vi "count_r2.vi"() -> ()   [LabVIEW 2015]
uses:
  <vilib>/myRIO/Instrument Drivers/Onboard IO/PWM/typedefs/PWM Reference.ctl
  <vilib>/myRIO/Common/Instrument Driver Framework/Utilities/typedefs/myRIO Generic Hardware Reference.ctl
  <vilib>/myRIO/Common/Instrument Driver Framework/Utilities/typedefs/Hardware Version Enum.ctl
  <vilib>/myRIO/Common/Instrument Driver Framework/Utilities/typedefs/myRIO v1.0 Reference.ctl
  <vilib>/myRIO/Common/Instrument Driver Framework/Utilities/typedefs/Generic FPGA Reference.ctl
  <vilib>/myRIO/Common/Instrument Driver Framework/myRIO v1.0/PWM/typedefs/PWM Channels Enum.ctl
  <vilib>/myRIO/Instrument Drivers/Onboard IO/PWM/typedefs/PWM Configuration.ctl
  <vilib>/userdefined/High Color/nirio_resource_hc.ctl
  <vilib>/myRIO/Common/Instrument Driver Framework/myRIO v1.0/PWM/vis/myRIO v1.1 Open PWM.vi
  <vilib>/myRIO/Common/Instrument Driver Framework/Utilities/vis/Validate Channels.vi
  <vilib>/myRIO/Common/Instrument Driver Framework/myRIO v1.0/PWM/vis/myRIO v1.0 Reserve PWM.vi
  <vilib>/myRIO/Instrument Drivers/Onboard IO/PWM/vis/Set Duty Cycle and Frequency.vi
  <vilib>/myRIO/Common/Instrument Driver Framework/myRIO v1.0/PWM/vis/myRIO v1.0 Build MUX Configuration PWM.vi
  <vilib>/myRIO/Common/Instrument Driver Framework/myRIO v1.0/Resource Manager/vis/myRIO v1.0 Reserve Channel List.vi
  <vilib>/myRIO/Common/Instrument Driver Framework/myRIO v1.0/Resource Manager/vis/myRIO v1.0 Create Configuration List.vi
  <vilib>/myRIO/Common/Instrument Driver Framework/myRIO v1.0/Resource Manager/vis/myRIO v1.0 Reserve Channel.vi
  <vilib>/myRIO/Common/Instrument Driver Framework/myRIO v1.0/Resource Manager/vis/myRIO v1.0 Unreserve Channel.vi
  <vilib>/myRIO/Common/Instrument Driver Framework/myRIO v1.0/Resource Manager/vis/myRIO v1.0 Build Mutex Name.vi
  <vilib>/FPGAPlugInAG/myRIO-1900/niLvFpga_Open_myRIO-1900.vi
  <vilib>/rvi/interface/common/dynamic/niFpgaDynamicAddResources.vi
  <vilib>/myRIO/Common/Instrument Driver Framework/Utilities/vis/FPGA Ref Manager.vi
  <vilib>/Utility/error.llb/Error Cluster From Error Code.vi
  <vilib>/myRIO/Common/Instrument Driver Framework/Utilities/vis/Ref Counter.vi
  <vilib>/rvi/errors/niLvFpgaAdjustHostInterfaceError.vi
  <vilib>/Utility/VariantDataType/GetNumericInfo.vi
  <vilib>/myRIO/Common/Instrument Driver Framework/myRIO v1.0/myRIO v1.1 Open.vi
  <vilib>/myRIO/Common/Instrument Driver Framework/Utilities/vis/IO Manager.vi
  <vilib>/myRIO/Common/Instrument Driver Framework/Utilities/vis/Configuration Manager.vi
  <vilib>/myRIO/Common/Instrument Driver Framework/myRIO v1.0/Resource Manager/vis/myRIO v1.0 Configure IO.vi
  <vilib>/myRIO/Common/Instrument Driver Framework/myRIO v1.0/myRIO v1.0 Close.vi
  <vilib>/myRIO/Common/Instrument Driver Framework/myRIO v1.0/PWM/vis/myRIO v1.0 Write PWM.vi
  <vilib>/rvi/interface/nirviOpenFPGA/nirviOpenFPGA.xnode
  FPGA Bitfiles/NavigationProjec_FPGATarget2_FPGAMainNavigati_PWPHW8gwDxI.lvbitx
  <vilib>/rvi/interface/nirviReadWriteControl/nirviReadWriteControl.xnode
  <vilib>/myRIO/Instrument Drivers/Onboard IO/PWM/vis/myRIO PWM Open.xnode
  <vilib>/myRIO/Instrument Drivers/Onboard IO/PWM/PWM.lvlib
  <vilib>/myRIO/Instrument Drivers/Utilities/Utilities.lvlib
  NiFpgaLv.dll
  <vilib>/rvi/interface/Simulation/niFpgaSimulationCallBeginRW.vi
panel:
  out "X Pos Lin Estimate":dbl
  out "Delta Lin Distance (ft)":dbl
  out "X Position Estimate":dbl
  out "Delta Distance (ft)":dbl
  out "heading degrees":dbl
  out "avg 456":dbl
  out "avg 123":dbl
  out "y position":dbl
  out "x position":dbl
  in  "start y":dbl=3.0
  in  "start x":dbl=1.0
  out "Delta Encoder Array":u32[](array[numeric])
  out "Robot Heading":dbl
  out "Current Encoder Array":u32[](array[numeric])
  out "Initial Encoder Array":u32[](array[numeric])
  in  "Encoder Reset":bool
  in  "master motor on switch":bool
  out "L Min Linear Velocity (ft/s) 2":dbl
  out "R Min Linear Velocity (ft/s)  2":dbl
  in  "Goal Y":dbl=3.0 format="%#_13g"
  in  "Goal X":dbl=20.0 format="%#_13g"
  out "x+y":dbl
  out "SYS.SELECTA":u8 format="%08b"
  out "ENC.B_c.CNTR":i32
  out "ENC.B_b.CNTR":i32
  out "ENC.B_a.CNTR":i32
  out "ENC.A_c.CNTR":i32
  out "ENC.A_b.CNTR":i32
  out "ENC.A_a.CNTR":i32
  out "Boolean":bool
  in  "R Desired Input Velocity (ft/s) 2":dbl(knob) scale=-4.0..4.0
  in  "front enable":bool
  in  "mid enable":bool
  in  "Rear enable":bool
  in  "Sync L -> R":bool
  in  "R Min Linear Velocity (ft/s)":dbl=-2.0 format="%#_13g"
  in  "R Max Linear Velocity (ft/s)":dbl=2.0 format="%#_13g"
  out "Rotational Velocity (RPS)":dbl
  in  "L Min Linear Velocity (ft/s)":dbl=-2.0 format="%#_13g"
  in  "L Max Linear Velocity (ft/s)":dbl=2.0 format="%#_13g"
  out "Current Rot Velocity (rot/s)":T1(graph)
  in  "L Desired Input Velocity (ft/s)":dbl(knob) scale=-4.0..4.0
  # "Motor Control Parameters"
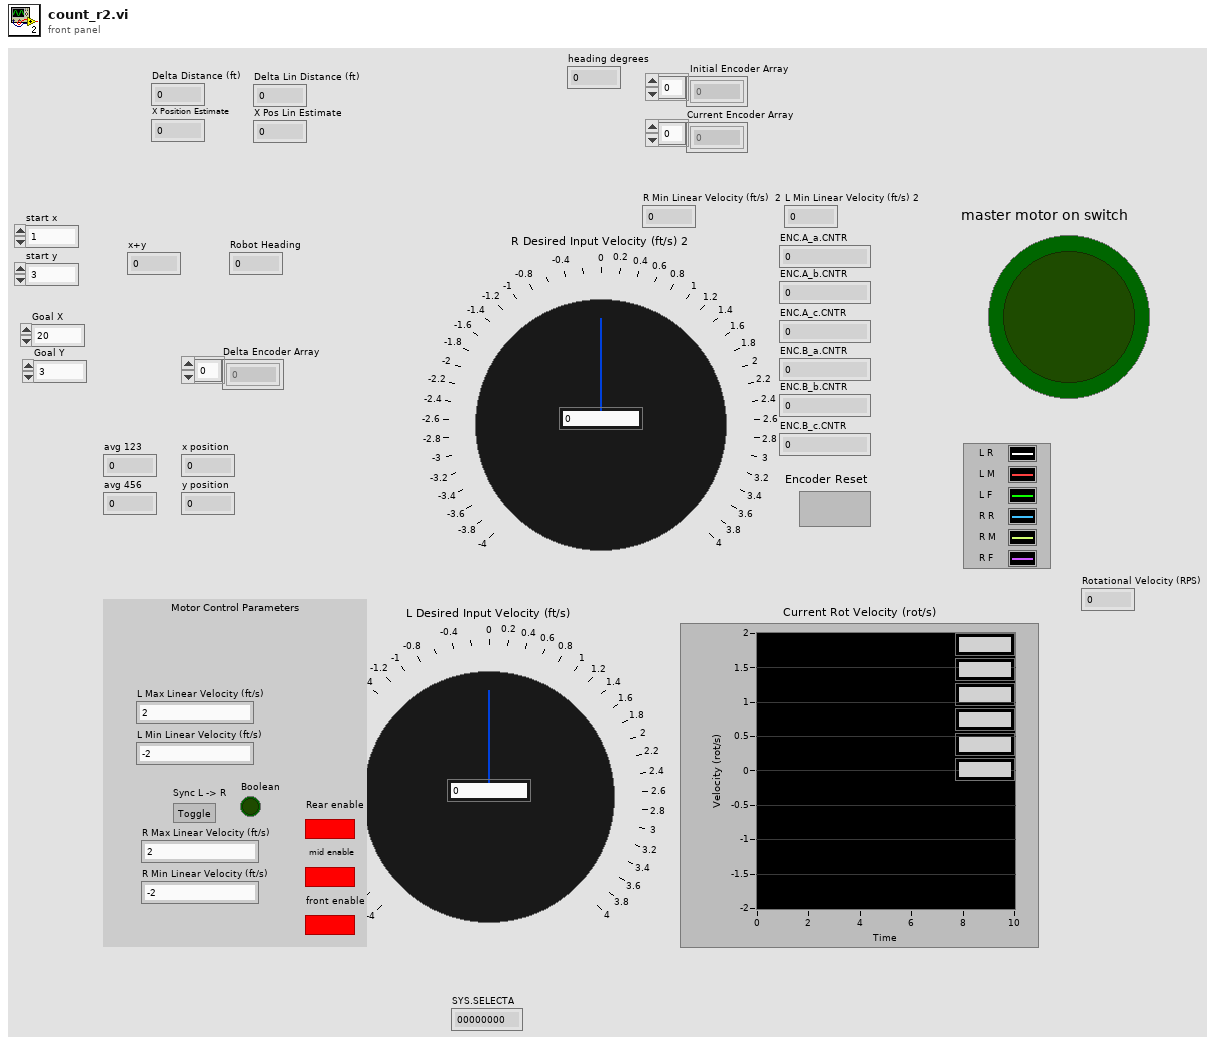
[diagram p1: front panel]
types:
  T1 = cluster{"Rotational Velocity (RPS)":dbl, "Rotational Velocity (RPS)":dbl, "Rotational Velocity (RPS)":dbl, "Rotational Velocity (RPS)":dbl, "Rotational Velocity (RPS)":dbl, "Rotational Velocity (RPS)":dbl}
  T2 = typedef "nirio_resource_hc.ctl" = tag
  T3 = typedef "Hardware Version Enum.ctl" = enum16{"Unknown", "myRIO-1900", "myRIO-1950", "roboRIO"}
  T4 = typedef "PWM.lvlib/PWM Reference.ctl" = cluster{"myRIO Reference":T5, "PWM Channels Enum":T8, "PWM Configuration":T9}
  T5 = typedef "myRIO Generic Hardware Reference.ctl" = cluster{"myRIO Model":T3, "myRIO Hardware Reference":T6}
  T6 = typedef "myRIO v1.0 Reference.ctl" = cluster{"Generic FPGA Reference":T7, "Allow multiple opens":bool}
  T7 = typedef "Generic FPGA Reference.ctl" = refnum<k20>
  T8 = typedef "PWM Channels Enum.ctl" = enum16{"Not Connected", "C/PWM0", "C/PWM1", "A/PWM0", "A/PWM1", "A/PWM2", "B/PWM0", "B/PWM1", "B/PWM2", "PWM/PWM0", "PWM/PWM1", "PWM/PWM2", "PWM/PWM3", "PWM/PWM4", "PWM/PWM5", "PWM/PWM6", "PWM/PWM7", "PWM/PWM8", "PWM/PWM9"}
  T9 = typedef "PWM.lvlib/PWM Configuration.ctl" = cluster{"Frequency":dbl, "Duty Cycle":dbl}
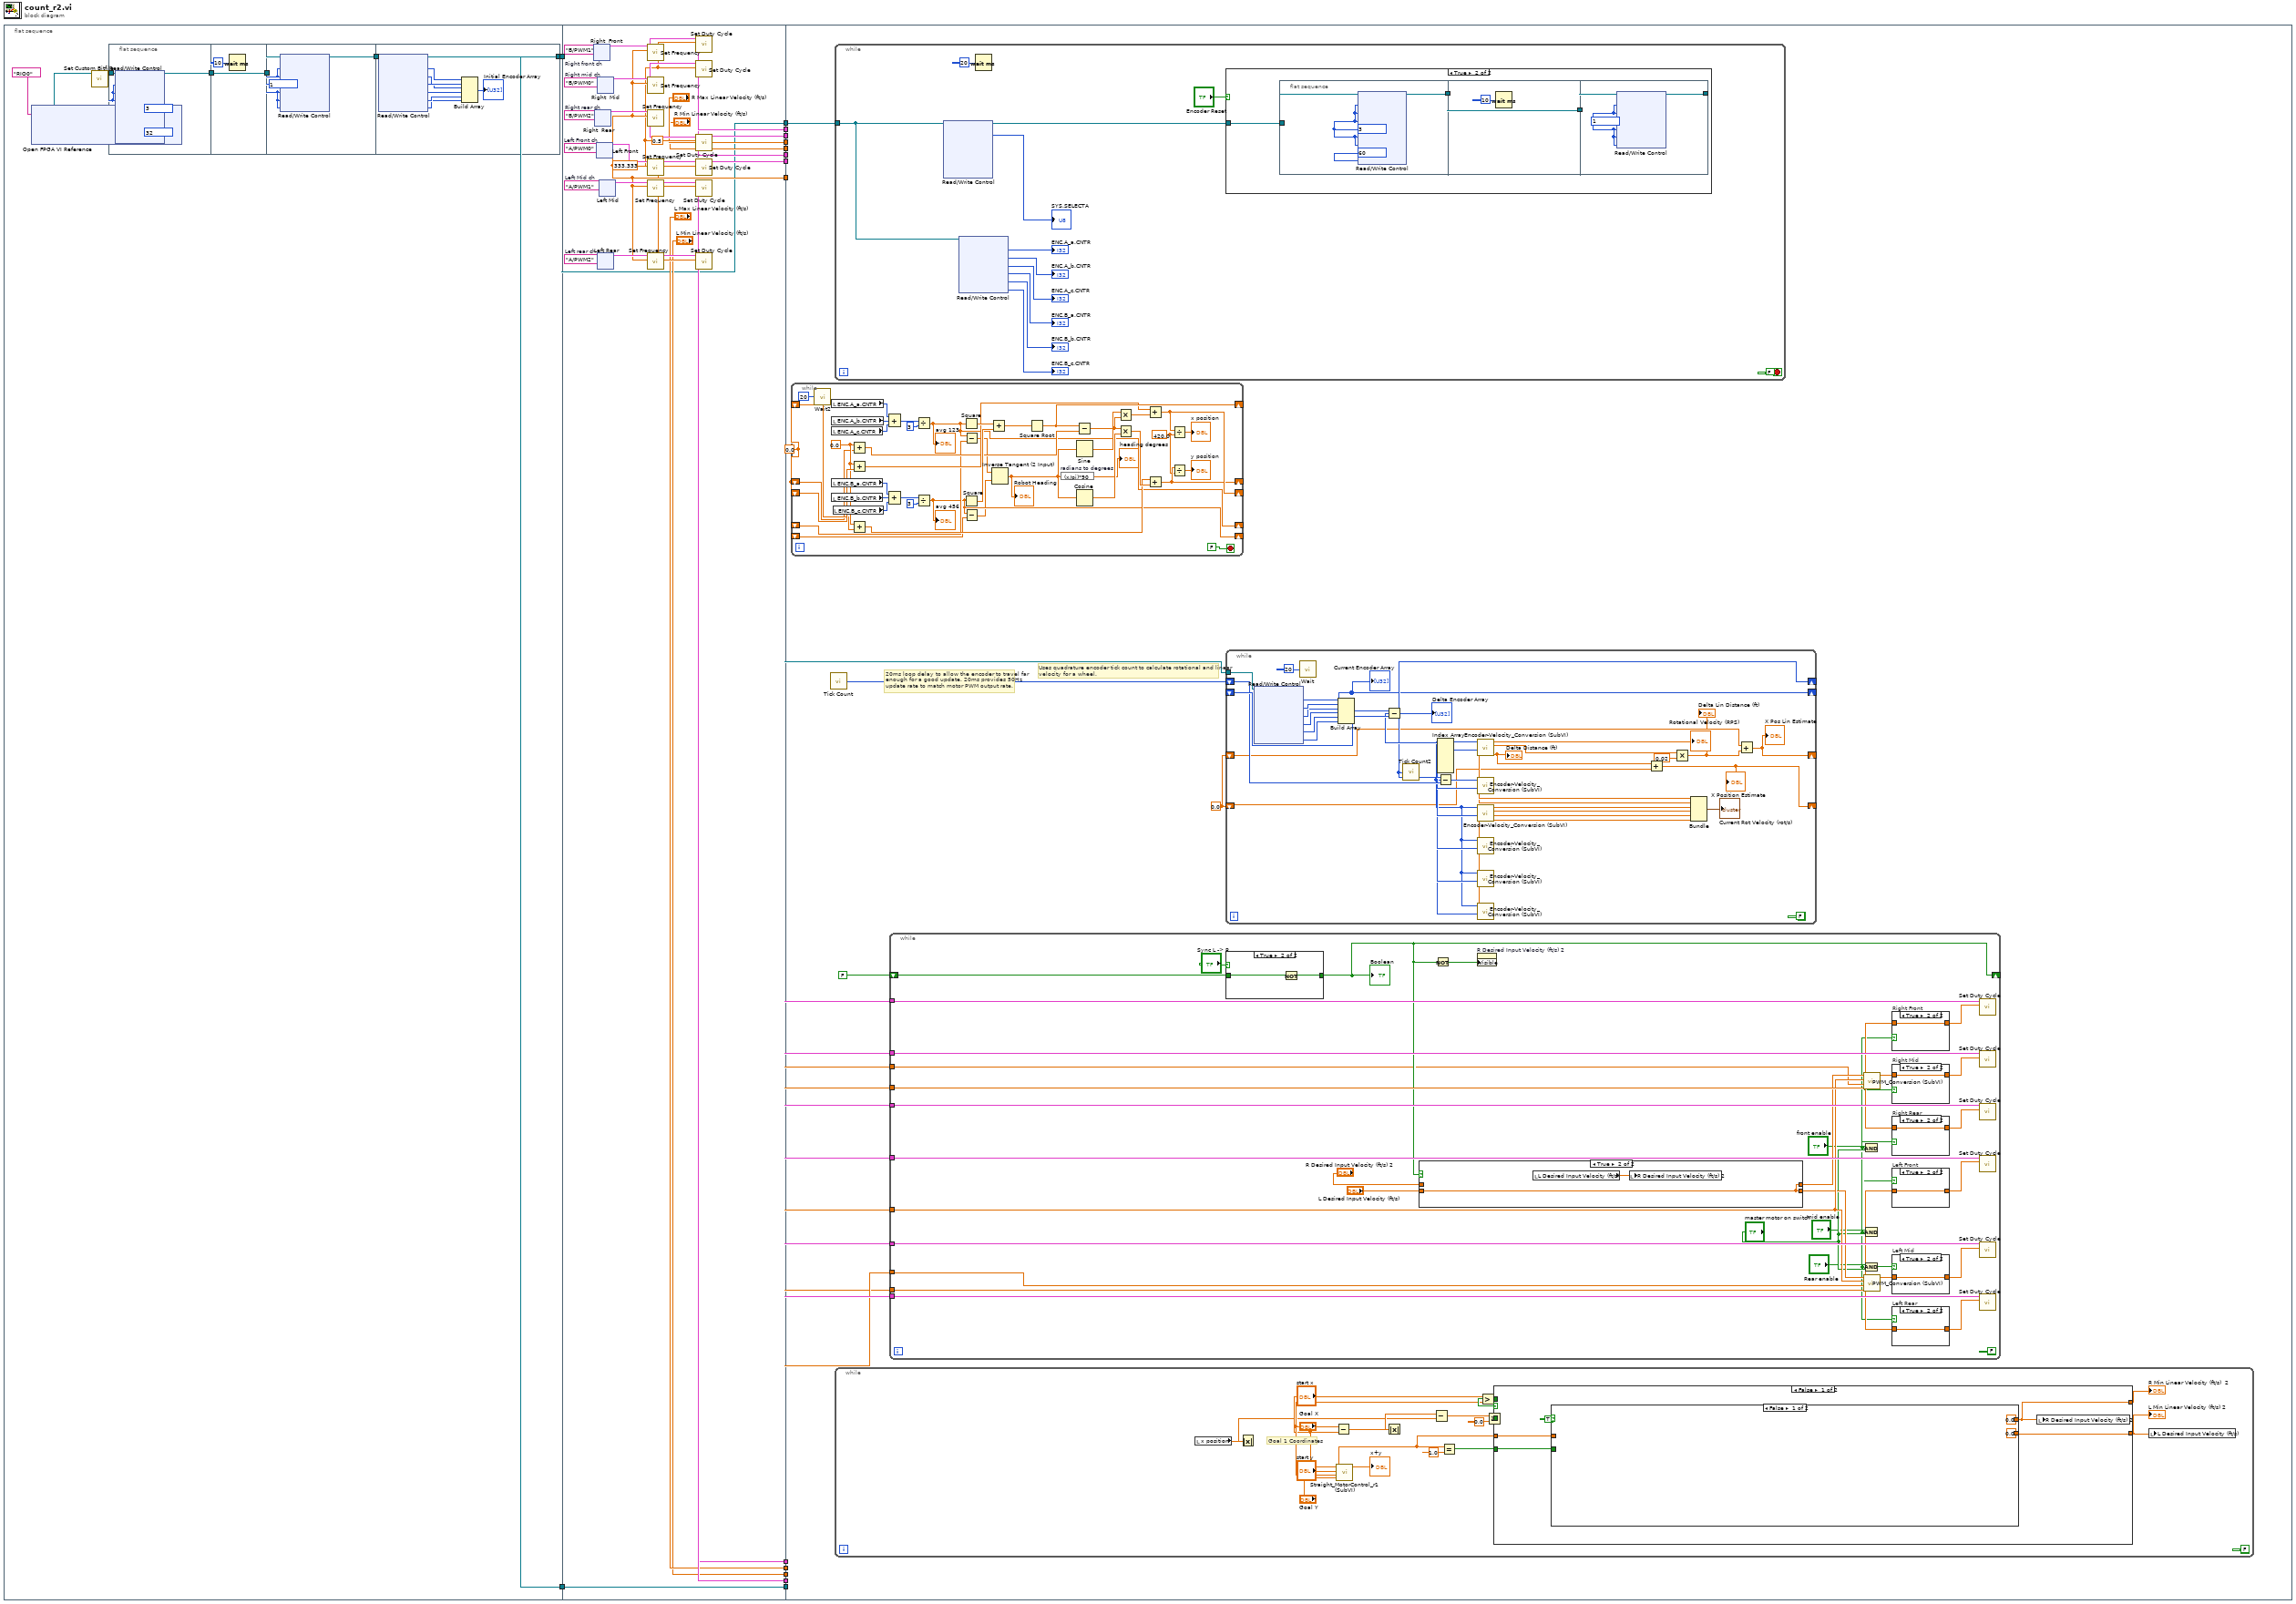
[diagram p0: block diagram]
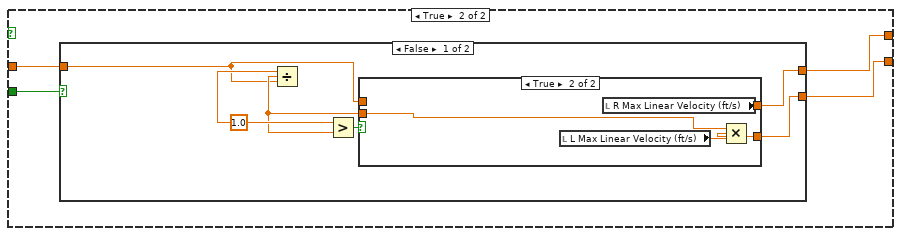
[diagram p2: hidden frame]
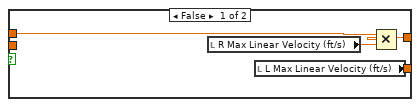
[diagram p3: hidden frame]
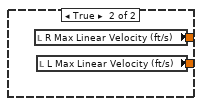
[diagram p4: hidden frame]
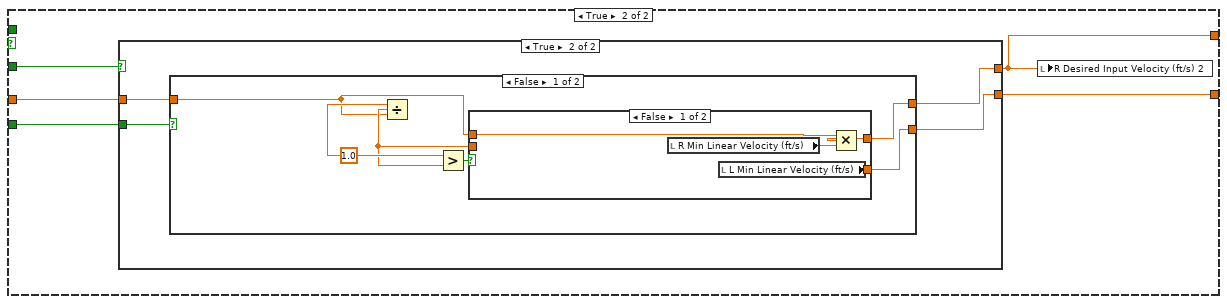
[diagram p5: hidden frame]
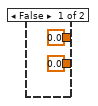
[diagram p6: hidden frame]
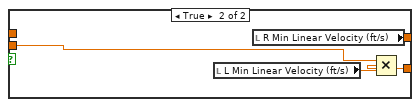
[diagram p7: hidden frame]
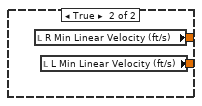
[diagram p8: hidden frame]
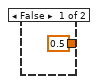
[diagram p11: hidden frame]
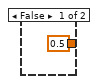
[diagram p12: hidden frame]
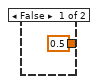
[diagram p13: hidden frame]
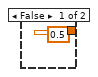
[diagram p14: hidden frame]
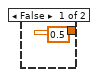
[diagram p15: hidden frame]
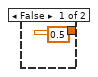
[diagram p16: hidden frame]
diagram:
  n1 = flat-sequence {
    tunnel: [w19] -> w3
    tunnel: [w19] -> w1
    tunnel: [w60] -> w15
    tunnel: [w55] -> w14
    tunnel: [w51] -> w13
    tunnel: [w50] -> w12
    tunnel: [w49] -> w11
    tunnel: [w48] -> w10
    tunnel: [w47] -> w9
    tunnel: ["L Max Linear Velocity (ft/s)"] -> w8
    tunnel: ["L Min Linear Velocity (ft/s)"] -> w7
    tunnel: ["R Max Linear Velocity (ft/s)"] -> w6
    tunnel: ["R Min Linear Velocity (ft/s)"] -> w5
    tunnel: [w42] -> w4
    tunnel: w3 -> [w41]
    tunnel: [w41] -> w2
    tunnel: w1 -> [w42]
    tunnel: w15 -> [w184]
    tunnel: w14 -> [w183]
    tunnel: w13 -> [w182]
    tunnel: w12 -> [w181]
    tunnel: w11 -> [w180]
    tunnel: w10 -> [w179]
    tunnel: w9 -> [w178]
    tunnel: w8 -> [w177]
    tunnel: w7 -> [w176]
    tunnel: w6 -> [w175]
    tunnel: w5 -> [w174]
    tunnel: w4 -> [w172]
    tunnel: w2 -> [w171]
    frame #0 {
      n2 = xnode "Open FPGA VI Reference"("resource name"=tag "RIO0") -> ("FPGA VI Reference Out"=w17:refnum<k20>)  [unwired: 1 in, 1 out]
      n3 = call <vilib>:"Set Custom Bitfile.vi"("Custom FPGA Reference In"=w17) -> ("Custom FPGA Reference Out"=w20:refnum<k20>)  [unwired: 9 in, 1 out]
      n4 = flat-sequence {
        tunnel: w20 -> [w25]
        tunnel: [w23] -> w22
        tunnel: w22 -> [w27]
        tunnel: [w27] -> w21
        tunnel: w21 -> [w30]
        tunnel: [w29] -> w18
        tunnel: [w32] -> w19
        tunnel: w18 -> [w33]
        frame #0 {
          w24 = u8 32 ("SYS.SELECTA")
          w26 = u8 3 ("ENC.B_c.CNFG")
          n5 = xnode "Read/Write Control"("FPGA VI Reference In"=w25, "ENC.A_a.CNFG"=w26, "ENC.A_b.CNFG"=w26, "ENC.A_c.CNFG"=w26, "ENC.B_a.CNFG"=w26, "ENC.B_b.CNFG"=w26, "ENC.B_c.CNFG"=w26, "SYS.SELECTA"=w24, "SYS.SELECTB"=w24) -> ("FPGA VI Reference Out"=w23:refnum<k20>)  [unwired: 1 in, 1 out]
        }
        frame #1 {
          n6 = Wait (ms)(milliseconds to wait=u32 10) -> ()  [unwired: 1 out]
        }
        frame #2 {
          w31 = u8 1 ("ENC.B_c.CNFG")
          n7 = xnode "Read/Write Control"("FPGA VI Reference In"=w30, "ENC.A_a.CNFG"=w31, "ENC.A_b.CNFG"=w31, "ENC.A_c.CNFG"=w31, "ENC.B_a.CNFG"=w31, "ENC.B_b.CNFG"=w31, "ENC.B_c.CNFG"=w31) -> ("FPGA VI Reference Out"=w29:refnum<k20>)  [unwired: 1 in, 1 out]
        }
        frame #3 {
          n8 = xnode "Read/Write Control"("FPGA VI Reference In"=w33) -> ("FPGA VI Reference Out"=w32:refnum<k20>, "ENC.A_a.CNTR"=w40:u32, "ENC.A_b.CNTR"=w39:u32, "ENC.A_c.CNTR"=w38:u32, "ENC.B_a.CNTR"=w37:u32, "ENC.B_b.CNTR"=w36:u32, "ENC.B_c.CNTR"=w35:u32)  [unwired: 1 in, 1 out]
          n9 = Build Array(w40, w39, w38, w37, w36, w35) -> (→"Initial Encoder Array":u32[])
        }
      }
    }
    frame #1 {
      w52 = 0.5 ("Duty Cycle")
      w60 = 333.333 ("Frequency [Hz]")
      w67 = tag "B/PWM2"  # Right rear ch
      w68 = tag "B/PWM0"  # Right mid ch
      w69 = tag "B/PWM1"  # Right front ch
      w70 = tag "A/PWM2"  # Left rear ch
      w71 = tag "A/PWM0"  # Left Front ch
      w72 = tag "A/PWM1"  # Left Mid ch
      n10 = xnode "Right  Front"("Channel Name"=w69) -> ("PWM Ref Out"=w63:T4)  [unwired: 2 in, 1 out]
      n11 = xnode "Right  Rear"("Channel Name"=w67) -> ("PWM Ref Out"=w61:T4)  [unwired: 2 in, 1 out]
      n12 = xnode "Left Front"("Channel Name"=w71) -> ("PWM Ref Out"=w65:T4)  [unwired: 2 in, 1 out]
      n13 = xnode "Right  Mid"("Channel Name"=w68) -> ("PWM Ref Out"=w62:T4)  [unwired: 2 in, 1 out]
      n14 = xnode "Left Rear"("Channel Name"=w70) -> ("PWM Ref Out"=w64:T4)  [unwired: 2 in, 1 out]
      n15 = xnode "Left Mid"("Channel Name"=w72) -> ("PWM Ref Out"=w66:T4)  [unwired: 2 in, 1 out]
      n16 = call <vilib>:"Set Frequency.vi"("Frequency [Hz]"=w60, "PWM Ref In"=w63) -> ("PWM Ref Out"=w56:T4)  [unwired: 7 in, 1 out]
      n17 = call <vilib>:"Set Frequency.vi"("Frequency [Hz]"=w60, "PWM Ref In"=w62) -> ("PWM Ref Out"=w57:T4)  [unwired: 7 in, 1 out]
      n18 = call <vilib>:"Set Frequency.vi"("Frequency [Hz]"=w60, "PWM Ref In"=w61) -> ("PWM Ref Out"=w58:T4)  [unwired: 7 in, 1 out]
      n19 = call <vilib>:"Set Frequency.vi"("Frequency [Hz]"=w60, "PWM Ref In"=w65) -> ("PWM Ref Out"=w53:T4)  [unwired: 7 in, 1 out]
      n20 = call <vilib>:"Set Frequency.vi"("Frequency [Hz]"=w60, "PWM Ref In"=w66) -> ("PWM Ref Out"=w59:T4)  [unwired: 7 in, 1 out]
      n21 = call <vilib>:"Set Frequency.vi"("Frequency [Hz]"=w60, "PWM Ref In"=w64) -> ("PWM Ref Out"=w54:T4)  [unwired: 7 in, 1 out]
      n22 = call <vilib>:"Set Duty Cycle.vi"("Duty Cycle"=w52, "PWM Ref In"=w56) -> ("PWM Ref Out"=w51:T4)  [unwired: 7 in, 1 out]
      n23 = call <vilib>:"Set Duty Cycle.vi"("Duty Cycle"=w52, "PWM Ref In"=w57) -> ("PWM Ref Out"=w50:T4)  [unwired: 7 in, 1 out]
      n24 = call <vilib>:"Set Duty Cycle.vi"("Duty Cycle"=w52, "PWM Ref In"=w58) -> ("PWM Ref Out"=w49:T4)  [unwired: 7 in, 1 out]
      n25 = call <vilib>:"Set Duty Cycle.vi"("Duty Cycle"=w52, "PWM Ref In"=w53) -> ("PWM Ref Out"=w48:T4)  [unwired: 7 in, 1 out]
      n26 = call <vilib>:"Set Duty Cycle.vi"("Duty Cycle"=w52, "PWM Ref In"=w59) -> ("PWM Ref Out"=w47:T4)  [unwired: 7 in, 1 out]
      n27 = call <vilib>:"Set Duty Cycle.vi"("Duty Cycle"=w52, "PWM Ref In"=w54) -> ("PWM Ref Out"=w55:T4)  [unwired: 7 in, 1 out]
    }
    frame #2 {
      w169 = 0.0
      w170 = 0.0
      # "Uses quadrature encoder tick count to calculate rotational and linear velocity for a wheel."
      # "20ms loop delay to allow the encoder to travel far enough for a good update. 20ms provides 50Hz update rate to match motor PWM output rate."
      n28 = while {
        shift-right: [w220] -> _
        shift-left: w170 -> [w188]
        shift-right: [w214] -> _
        shift-left: w170 -> [w199]
        shift-right: [w212] -> _
        shift-left: w170 -> [w187]
        shift-right: [w191] -> _
        shift-left: _ -> [w194]
        shift-right: [w192] -> _
        shift-left: _ -> [w193]
        stop <- FALSE stop-if-true
        w197 = 0.0
        w211 = 420.0 ("y")
        n29 = call "Wait2"("Count(mSec)"=u32 20) -> ()  [unwired: 1 out]
        n30 = local read "ENC.A_a.CNTR"() -> (w205:i32)
        n31 = local read "ENC.A_b.CNTR"() -> (w204:i32)
        n32 = local read "ENC.A_c.CNTR"() -> (w203:i32)
        n33 = local read "ENC.B_a.CNTR"() -> (w202:i32)
        n34 = local read "ENC.B_b.CNTR"() -> (w201:i32)
        n35 = local read "ENC.B_c.CNTR"() -> (w200:i32)
        n36 = Add(x=w197, y=w187) -> (x+y=w195:dbl)
        n37 = Add(x=w197, y=w199) -> (x+y=w198:dbl)
        n38 = Add(x=w197, y=w188) -> (x+y=w196:dbl)
        n39 = Compound Arithmetic op=ADD(w205, w204, w203) -> (w216:i32)
        n40 = Compound Arithmetic op=ADD(w202, w201, w200) -> (w215:i32)
        n41 = Divide(x=w216, y=3) -> (x/y=w191:dbl)
        "avg 123" <- w191
        n42 = Divide(x=w215, y=3) -> (x/y=w192:dbl)
        "avg 456" <- w192
        n43 = Square(x=w191) -> (x^2=w223:dbl)
        n44 = Square(x=w192) -> (x^2=w225:dbl)
        n45 = Subtract(x=w191, y=w194) -> (x-y=w190:dbl)
        n46 = Subtract(x=w192, y=w193) -> (x-y=w189:dbl)
        n47 = Add(x=w223, y=w225) -> (x+y=w226:dbl)
        n48 = Inverse Tangent (2 Input)(1:w189, 2:w190) -> (0:w209:dbl)
        "Robot Heading" <- w209
        n49 = Square Root(x=w226) -> (sqrt(x)=w220:dbl)
        n50 = expression code="(x/pi)*90" "radians to degrees"(w209) -> (→"heading degrees":dbl)
        n51 = Subtract(x=w220, y=w195) -> (x-y=w219:dbl)
        n52 = Sine(x=w209) -> (sin(x)=w222:dbl)
        n53 = Cosine(x=w209) -> (cos(x)=w221:dbl)
        n54 = Multiply(x=w222, y=w219) -> (x*y=w218:dbl)
        n55 = Multiply(x=w219, y=w221) -> (x*y=w217:dbl)
        n56 = Add(x=w198, y=w218) -> (x+y=w214:dbl)
        n57 = Add(x=w196, y=w217) -> (x+y=w212:dbl)
        n58 = Divide(x=w214, y=w211) -> (x/y=→"x position":dbl)
        n59 = Divide(x=w212, y=w211) -> (x/y=→"y position":dbl)
      }
      n60 = call "Tick Count"() -> ("Tick Count(uSec)"=w185:u32)
      n61 = while {
        tunnel: w172 -> [w302]
        stop <- FALSE stop-if-true
        n62 = xnode "Read/Write Control"("FPGA VI Reference In"=w302) -> ("FPGA VI Reference Out"=w300:refnum<k20>, "SYS.SELECTA"=→"SYS.SELECTA":u8)  [unwired: 1 in, 6 out]
        n63 = xnode "Read/Write Control"("FPGA VI Reference In"=w302) -> ("ENC.A_a.CNTR"=→"ENC.A_a.CNTR":u32, "ENC.A_b.CNTR"=→"ENC.A_b.CNTR":u32, "ENC.A_c.CNTR"=→"ENC.A_c.CNTR":u32, "ENC.B_a.CNTR"=→"ENC.B_a.CNTR":u32, "ENC.B_b.CNTR"=→"ENC.B_b.CNTR":u32, "ENC.B_c.CNTR"=→"ENC.B_c.CNTR":u32)  [unwired: 1 in, 2 out]
        n64 = Wait (ms)(milliseconds to wait=u32 20) -> ()  [unwired: 1 out]
        n65 = case shown="True" "Encoder Reset" {
          tunnel: w300 -> [_ w311]
          frame False {
          }
          frame True {
            n66 = flat-sequence {
              tunnel: w311 -> [w316]
              tunnel: [w314] -> w313
              tunnel: w313 -> [w318]
              tunnel: [w318] -> w312
              tunnel: w312 -> [w321]
              tunnel: [w320] -> _
              frame #0 {
                w315 = u8 60 ("SYS.SELECTA")
                w317 = u8 3 ("ENC.B_c.CNFG")
                n67 = xnode "Read/Write Control"("FPGA VI Reference In"=w316, "ENC.A_a.CNFG"=w317, "ENC.A_b.CNFG"=w317, "ENC.A_c.CNFG"=w317, "ENC.B_a.CNFG"=w317, "ENC.B_b.CNFG"=w317, "ENC.B_c.CNFG"=w317, "SYS.SELECTA"=w315, "SYS.SELECTB"=w315) -> ("FPGA VI Reference Out"=w314:refnum<k20>)  [unwired: 1 in, 1 out]
              }
              frame #1 {
                n68 = Wait (ms)(milliseconds to wait=u32 10) -> ()  [unwired: 1 out]
              }
              frame #2 {
                w322 = u8 1 ("ENC.B_c.CNFG")
                n69 = xnode "Read/Write Control"("FPGA VI Reference In"=w321, "ENC.A_a.CNFG"=w322, "ENC.A_b.CNFG"=w322, "ENC.A_c.CNFG"=w322, "ENC.B_a.CNFG"=w322, "ENC.B_b.CNFG"=w322, "ENC.B_c.CNFG"=w322) -> ("FPGA VI Reference Out"=w320:refnum<k20>)  [unwired: 1 in, 1 out]
              }
            }
          }
        }
      }
      n70 = while {
        stop <- FALSE stop-if-true
        # "Goal 1 Coordinates"
        n71 = local read "x position"() -> (w234:dbl)
        n72 = Absolute Value(x=w234) -> (abs(x)=w228:dbl)
        n73 = Subtract(x="Goal X", y="start x") -> (x-y=w230:dbl)
        n74 = call "Straight_MotorControl_r1 (SubVI).vi"("Goal Y Coord"="Goal Y", "Goal X Coord"="Goal X", "Current Y Pos"="start y", "Current X Pos"="start x") -> ("Numeric Out Y"=w244:dbl)  [unwired: 7 in]
        "x+y" <- w244
        n75 = Absolute Value(x=w230) -> (abs(x)=w229:dbl)
        n76 = Subtract(x=w229, y=w228) -> (x-y=w227:dbl)
        n77 = Equal?(x=w244, y=1.0) -> (x = y?=w242:bool)
        n78 = Greater?(x="start x", y="Goal X") -> (0:w233:bool)
        n79 = Greater Or Equal?(x=w227, y=0.0) -> (x >= y?=w235:bool)
        n80 = case shown="False" w233 {
          tunnel: w244 -> [w247 w276]
          tunnel: w242 -> [w246 w275]
          tunnel: [w249 w274] -> w240
          tunnel: [w248 w273] -> w239
          tunnel: w235 -> [_ w272]
          tunnel: w233 -> [_ _]
          frame False {
            n81 = case shown="False" TRUE {
              tunnel: w247 -> [_ w255]
              tunnel: w246 -> [_ w254]
              tunnel: [0.0 ("R Min Linear Velocity (ft/s)") w253] -> w249
              tunnel: [0.0 ("L Min Linear Velocity (ft/s)") w252] -> w248
              frame False {
              }
              frame True {
                n82 = case shown="False" w254 {
                  tunnel: [w258 w270] -> w252
                  tunnel: [w257 w271] -> w253
                  tunnel: w255 -> [w256 _]
                  frame False {
                    w261 = 1.0 ("x")
                    n83 = Divide(x=w261, y=w256) -> (x/y=w260:dbl)
                    n84 = Greater?(x=w261, y=w260) -> (0:w259:bool)
                    n85 = case shown="True" w259 {
                      tunnel: w260 -> [_ w269]
                      tunnel: [w262 w267] -> w258
                      tunnel: [w263 w266] -> w257
                      tunnel: w256 -> [w265 _]
                      frame False {
                        n86 = local read "R Max Linear Velocity (ft/s)"() -> (w264:dbl)
                        n87 = local read "L Max Linear Velocity (ft/s)"() -> (w262:dbl)
                        n88 = Multiply(x=w265, y=w264) -> (x*y=w263:dbl)
                      }
                      frame True {
                        n89 = local read "L Max Linear Velocity (ft/s)"() -> (w268:dbl)
                        n90 = local read "R Max Linear Velocity (ft/s)"() -> (w266:dbl)
                        n91 = Multiply(x=w269, y=w268) -> (x*y=w267:dbl)
                      }
                    }
                  }
                  frame True {
                    n92 = local read "R Max Linear Velocity (ft/s)"() -> (w271:dbl)
                    n93 = local read "L Max Linear Velocity (ft/s)"() -> (w270:dbl)
                  }
                }
              }
            }
            n94 = local write "R Desired Input Velocity (ft/s) 2"(w249) -> ()
          }
          frame True {
            n95 = case shown="True" w272 {
              tunnel: w276 -> [_ w282]
              tunnel: w275 -> [_ w281]
              tunnel: [0.0 ("R Min Linear Velocity (ft/s)") w280] -> w274
              tunnel: [0.0 ("L Min Linear Velocity (ft/s)") w279] -> w273
              frame False {
              }
              frame True {
                n96 = case shown="False" w281 {
                  tunnel: [w285 w297] -> w279
                  tunnel: [w284 w298] -> w280
                  tunnel: w282 -> [w283 _]
                  frame False {
                    w288 = 1.0 ("x")
                    n97 = Divide(x=w288, y=w283) -> (x/y=w287:dbl)
                    n98 = Greater?(x=w288, y=w287) -> (0:w286:bool)
                    n99 = case shown="False" w286 {
                      tunnel: w287 -> [_ w296]
                      tunnel: [w289 w294] -> w285
                      tunnel: [w290 w293] -> w284
                      tunnel: w283 -> [w292 _]
                      frame False {
                        n100 = local read "R Min Linear Velocity (ft/s)"() -> (w291:dbl)
                        n101 = local read "L Min Linear Velocity (ft/s)"() -> (w289:dbl)
                        n102 = Multiply(x=w292, y=w291) -> (x*y=w290:dbl)
                      }
                      frame True {
                        n103 = local read "L Min Linear Velocity (ft/s)"() -> (w295:dbl)
                        n104 = local read "R Min Linear Velocity (ft/s)"() -> (w293:dbl)
                        n105 = Multiply(x=w296, y=w295) -> (x*y=w294:dbl)
                      }
                    }
                  }
                  frame True {
                    n106 = local read "R Min Linear Velocity (ft/s)"() -> (w298:dbl)
                    n107 = local read "L Min Linear Velocity (ft/s)"() -> (w297:dbl)
                  }
                }
              }
            }
            n108 = local write "R Desired Input Velocity (ft/s) 2"(w274) -> ()
          }
        }
        "R Min Linear Velocity (ft/s)  2" <- w240
        "L Min Linear Velocity (ft/s) 2" <- w239
        n109 = local write "L Desired Input Velocity (ft/s)"(w239) -> ()
      }
      n110 = while {
        tunnel: w184 -> [w341]
        tunnel: w183 -> [w351]
        tunnel: w182 -> [w356]
        tunnel: w181 -> [w355]
        tunnel: w180 -> [w354]
        tunnel: w179 -> [w353]
        tunnel: w178 -> [w352]
        tunnel: w177 -> [w344]
        tunnel: w176 -> [w343]
        tunnel: w175 -> [w330]
        tunnel: w174 -> [w342]
        shift-right: [w331] -> _
        shift-left: FALSE -> [w332]
        stop <- FALSE stop-if-true
        n111 = case shown="True" "Sync L -> R" {
          tunnel: w332 -> [w358 w360]
          tunnel: [w358 w359] -> w331
          frame False {
          }
          frame True {
            n112 = Not(x=w360) -> (.not. x?=w359:bool)
          }
        }
        "Boolean" <- w331
        n113 = case shown="True" w331 {
          tunnel: "L Desired Input Velocity (ft/s)" -> [w374 w375]
          tunnel: [w374 w375] -> w337
          tunnel: "R Desired Input Velocity (ft/s) 2" -> [w373 _]
          tunnel: [w373 w375] -> w335
          frame False {
          }
          frame True {
            n114 = local read "L Desired Input Velocity (ft/s)"() -> (w376:dbl)
            n115 = local write "R Desired Input Velocity (ft/s) 2"(w376) -> ()
          }
        }
        n116 = Not(x=w331) -> (.not. x?=w334:bool)
        n117 = property on="R Desired Input Velocity (ft/s) 2" class="Knob (strict)"("Visible"=w334) -> ()  [unwired: 2 in, 2 out]
        n118 = call "PWM_Conversion (SubVI).vi"("Min Linear Velocity (ft/s)"=w342, "Max Linear Velocity (ft/s)"=w330, "PWM Frequency"=w341, "Linear Velocity Input (ft/s)"=w335) -> ("PWM Signal Output"=w339:dbl)  [unwired: 7 in]
        n119 = call "PWM_Conversion (SubVI).vi"("Min Linear Velocity (ft/s)"=w343, "Max Linear Velocity (ft/s)"=w344, "PWM Frequency"=w341, "Linear Velocity Input (ft/s)"=w337) -> ("PWM Signal Output"=w340:dbl)  [unwired: 7 in]
        n120 = Compound Arithmetic op=AND("front enable", "master motor on switch") -> (w324:bool)
        n121 = Compound Arithmetic op=AND("mid enable", "master motor on switch") -> (w323:bool)
        n122 = Compound Arithmetic op=AND("Rear enable", "master motor on switch") -> (w325:bool)
        n123 = case "Right Front" shown="True" w324 {
          tunnel: [0.5 w372] -> w345
          tunnel: w339 -> [_ w372]
          frame False {
          }
          frame True {
          }
        }
        n124 = case "Right Mid" shown="True" w323 {
          tunnel: [0.5 w370] -> w346
          tunnel: w339 -> [_ w370]
          frame False {
          }
          frame True {
          }
        }
        n125 = case "Right Rear" shown="True" w325 {
          tunnel: [0.5 w368] -> w347
          tunnel: w339 -> [_ w368]
          frame False {
          }
          frame True {
          }
        }
        n126 = case "Left Front" shown="True" w324 {
          tunnel: [0.5 w366] -> w348
          tunnel: w340 -> [_ w366]
          frame False {
          }
          frame True {
          }
        }
        n127 = case "Left Mid" shown="True" w323 {
          tunnel: [0.5 w364] -> w349
          tunnel: w340 -> [_ w364]
          frame False {
          }
          frame True {
          }
        }
        n128 = case "Left Rear" shown="True" w325 {
          tunnel: [0.5 w362] -> w350
          tunnel: w340 -> [_ w362]
          frame False {
          }
          frame True {
          }
        }
        n129 = call <vilib>:"Set Duty Cycle.vi"("Duty Cycle"=w345, "PWM Ref In"=w356) -> ()  [unwired: 7 in, 2 out]
        n130 = call <vilib>:"Set Duty Cycle.vi"("Duty Cycle"=w346, "PWM Ref In"=w355) -> ()  [unwired: 7 in, 2 out]
        n131 = call <vilib>:"Set Duty Cycle.vi"("Duty Cycle"=w347, "PWM Ref In"=w354) -> ()  [unwired: 7 in, 2 out]
        n132 = call <vilib>:"Set Duty Cycle.vi"("Duty Cycle"=w348, "PWM Ref In"=w353) -> ()  [unwired: 7 in, 2 out]
        n133 = call <vilib>:"Set Duty Cycle.vi"("Duty Cycle"=w349, "PWM Ref In"=w352) -> ()  [unwired: 7 in, 2 out]
        n134 = call <vilib>:"Set Duty Cycle.vi"("Duty Cycle"=w350, "PWM Ref In"=w351) -> ()  [unwired: 7 in, 2 out]
      }
      n135 = while {
        shift-right: [w385] -> _
        shift-left: _ -> [w403]
        shift-right: [w401] -> _
        shift-left: w185 -> [w400]
        tunnel: w171 -> [w410]
        shift-right: [w382] -> _
        shift-left: w169 -> [w383]
        shift-right: [w377] -> _
        shift-left: w169 -> [w379]
        stop <- FALSE stop-if-true
        n136 = xnode "Read/Write Control"("FPGA VI Reference In"=w410) -> ("ENC.A_a.CNTR"=w409:u32, "ENC.A_b.CNTR"=w408:u32, "ENC.A_c.CNTR"=w407:u32, "ENC.B_a.CNTR"=w406:u32, "ENC.B_b.CNTR"=w405:u32, "ENC.B_c.CNTR"=w404:u32)  [unwired: 1 in, 2 out]
        n137 = call "Wait"("Count(mSec)"=u32 20) -> ()  [unwired: 1 out]
        n138 = Build Array(w409, w408, w407, w406, w405, w404) -> (w385:u32[])
        "Current Encoder Array" <- w385
        n139 = Subtract(x=w385, y=w403) -> (x-y=w402:u32[])
        "Delta Encoder Array" <- w402
        n140 = call "Tick Count2"() -> ("Tick Count(uSec)"=w401:u32)
        n141 = Index Array(array=w402) -> (element #1=w399:u32, element #2=w398:u32, element #3=w397:u32, element #4=w396:u32, element #5=w395:u32, element #6=w394:u32)  [unwired: 6 in]
        n142 = Subtract(x=w401, y=w400) -> (x-y=w393:u32)
        n143 = call "Encoder-Velocity_Conversion (SubVI).vi"("delta  Encoder Count"=w399, "dt (uSec)"=w393) -> ("Distance (ft)"=w384:dbl, "Linear Velocity (ft/s)"=w381:dbl, "Rotational Velocity (RPS)"=w392:dbl)  [unwired: 7 in]
        "Rotational Velocity (RPS)" <- w392
        "Delta Distance (ft)" <- w384
        n144 = call "Encoder-Velocity_Conversion (SubVI).vi"("delta  Encoder Count"=w398, "dt (uSec)"=w393) -> ("Rotational Velocity (RPS)"=w391:dbl)  [unwired: 7 in, 2 out]
        n145 = call "Encoder-Velocity_Conversion (SubVI).vi"("delta  Encoder Count"=w397, "dt (uSec)"=w393) -> ("Rotational Velocity (RPS)"=w390:dbl)  [unwired: 7 in, 2 out]
        n146 = call "Encoder-Velocity_Conversion (SubVI).vi"("delta  Encoder Count"=w396, "dt (uSec)"=w393) -> ("Rotational Velocity (RPS)"=w389:dbl)  [unwired: 7 in, 2 out]
        n147 = call "Encoder-Velocity_Conversion (SubVI).vi"("delta  Encoder Count"=w395, "dt (uSec)"=w393) -> ("Rotational Velocity (RPS)"=w388:dbl)  [unwired: 7 in, 2 out]
        n148 = call "Encoder-Velocity_Conversion (SubVI).vi"("delta  Encoder Count"=w394, "dt (uSec)"=w393) -> ("Rotational Velocity (RPS)"=w387:dbl)  [unwired: 7 in, 2 out]
        n149 = Add(x=w384, y=w383) -> (x+y=w382:dbl)
        "X Position Estimate" <- w382
        n150 = Multiply(x=w381, y=0.02) -> (x*y=w378:dbl)
        "Delta Lin Distance (ft)" <- w378
        n151 = Bundle("Rotational Velocity (RPS)"=w392, "Rotational Velocity (RPS)"=w391, "Rotational Velocity (RPS)"=w390, "Rotational Velocity (RPS)"=w389, "Rotational Velocity (RPS)"=w388, "Rotational Velocity (RPS)"=w387) -> (→"Current Rot Velocity (rot/s)":T1)  [unwired: 1 in]
        n152 = Add(x=w379, y=w378) -> (x+y=w377:dbl)
        "X Pos Lin Estimate" <- w377
      }
    }
  }
